vi "TestMeasure.vi"(7 "Samples":i32=5, 8 "error in (no error)":errorcluster, 11 "communication":i16(ring)=2 items=["USB - Nova2", "USB - Vega", "USB - USBI", "RS232", "GPIB"]) -> (0 "error out":errorcluster, 1 "variance":dbl format="%.2e", 2 "std deviation":dbl format="%.2e", 3 "mean":dbl format="%.4f")   [LabVIEW 2012]
doc: "PowerDemo.vi\nThe Demo enables power measurement and display results.\nVersion 1.00\nLast Updated 16 Mars 2005\n\nDemo Program Steps:\n \n1) The vi executes InitCom.vi to open the communication session.\nThe default is RS232,Port2,9600 bps and Address 10 for USB.\n\nYou have to select USB or RS232 Protocol and\nupdate these values for any change.\n\n2) The vi executes ConfMeasure.vi to Send \"FP\" (Force Power) to Device and \"SI\" (Send unIts) to receive the units\n\n3) The vi executes a loop of SendPower.vi to get measurements.\nWhen no Overrange value the vi add value to array for update\nstatistics values.\n\nIn case of Error:\nError Out contains the Error Number and the vi's name where the error occured.\n\nVISA Error Codes -10738077360 to -1073807231\nOphir Error Codes -1300 to 1340"
uses:
  <vilib>/Analysis/NI_AALBase.lvlib
panel:
  out "mean 2":dbl
  out "Units":string
  in  "Set Wavelength":string="275"
  out "Device Response 2":string="\r\n"
  out "Device Response":string="\r\n"
  out "Overrange":bool
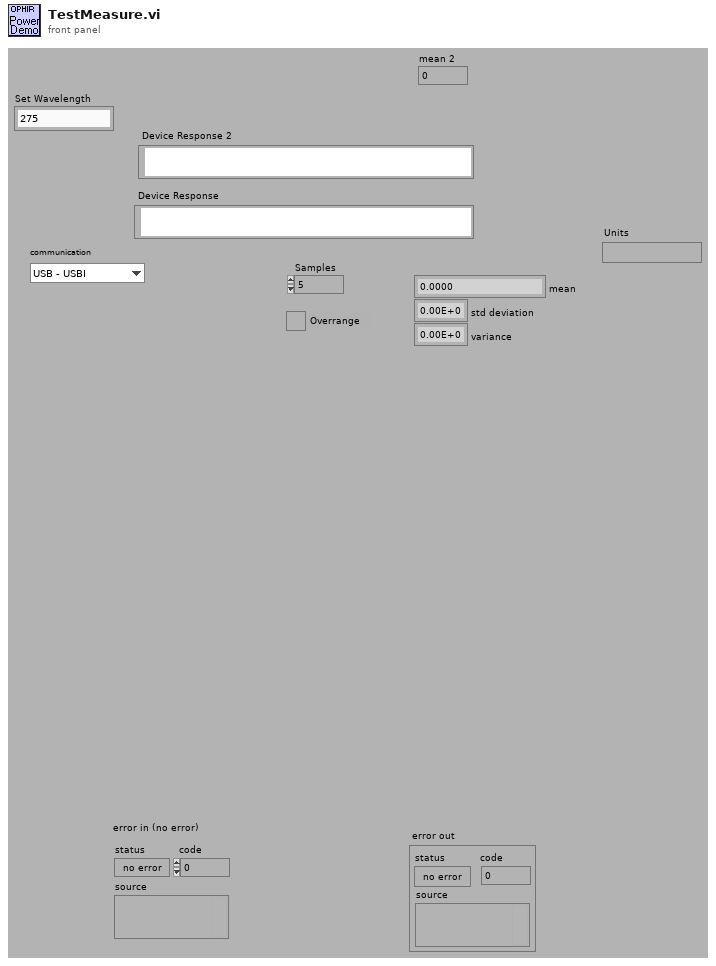
[diagram p1: front panel]
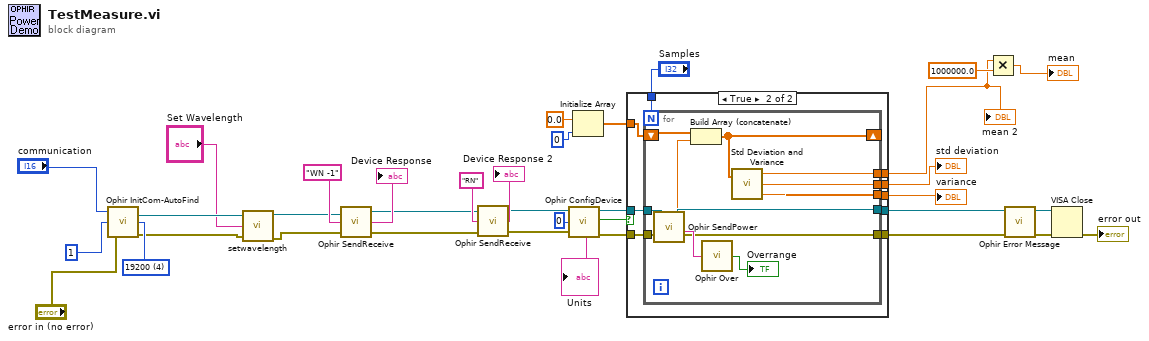
[diagram p0: block diagram]
diagram:
  w31 = i16 4 items=["300", "1200", "4800", "9600", "19200", "38400"] ("Baud Rate (3:9600)")
  n1 = call "Ophir InitCom-AutoFind.vi"("Baud Rate (3:9600)"=w31, "communication"="communication", "Port Number (default 2)"=i16 1, "error in (no error)"="error in (no error)") -> ("Dup Visa Session"=w7:refnum<visa-resource-name>, "error out"=w6:errorcluster)  [unwired: 2 out]
  n2 = call "setwavelength.vi"("Dup Visa Session"=w7, "Set Wavelength"="Set Wavelength", "error in (no error)"=w6) -> ("dup Visa Session"=w9:refnum<visa-resource-name>, "error out"=w8:errorcluster)  [unwired: 3 in]
  n3 = call "Ophir SendReceive.vi"("error in (no error)"=w8, "Command"="WN -1", "Visa Session"=w9) -> ("error out"=w11:errorcluster, "Frame Output"=→"Device Response":string, "dup Visa Session"=w13:refnum<visa-resource-name>)
  n4 = call "Ophir SendReceive.vi"("error in (no error)"=w11, "Command"="RN", "Visa Session"=w13) -> ("error out"=w10:errorcluster, "Frame Output"=→"Device Response 2":string, "dup Visa Session"=w12:refnum<visa-resource-name>)
  n5 = call "Ophir ConfigDevice.vi"("Visa Session"=w12, "Measure Choice (0:Power)"=u16 0, "error in (no error)"=w10) -> ("dup Visa Session"=w33:refnum<visa-resource-name>, "OK ?"=w34:bool, "Units"=→"Units":string, "error out"=w32:errorcluster)
  n6 = Initialize Array(0.0 ("element"), 0 ("dimension size")) -> (w21:dbl[])
  n7 = case shown="True" w34 {
    tunnel: w33 -> [w37 w47]
    tunnel: w32 -> [w38 w46]
    tunnel: [w37 w45] -> w28
    tunnel: [w38 w44] -> w25
    tunnel: "Samples" -> [_ w43]
    tunnel: w21 -> [_ w42]
    tunnel: [_ w41] -> w20
    tunnel: [_ w40] -> w19
    tunnel: [_ w39] -> w2
    frame False {
      # "Force Power Configuration failed"
    }
    frame True {
      n8 = for {
        N: w43 -> [_]
        tunnel: w47 -> [w59]
        tunnel: w46 -> [w58]
        tunnel: [w57] -> w45
        tunnel: [w54] -> w44
        shift-right: [w51] -> _
        shift-left: w42 -> [w53]
        tunnel: [w50] -> w39
        tunnel: [w49] -> w40
        tunnel: [w48] -> w41
        n9 = call "Ophir SendPower.vi"("Visa Session"=w59, "error in (no error)"=w58) -> ("dup Visa Session"=w57:refnum<visa-resource-name>, "Value Number"=w52:dbl, "Value String"=w56:string, "error out"=w54:errorcluster)
        n10 = Build Array (concatenate)(w53, w52) -> (w51:dbl[])
        n11 = call "Ophir Over.vi"("Value String"=w56) -> ("Overrange"=→"Overrange":bool)
        n12 = call <vilib>:"Std Deviation and Variance.vi"("X"=w51) -> ("mean"=w50:dbl, "standard deviation"=w49:dbl, "variance"=w48:dbl)  [unwired: 1 in]
      }
    }
  }
  "std deviation" <- w19
  "variance" <- w20
  "mean 2" <- w2
  n13 = Multiply(x=w2, y=1000000.0) -> (x*y=→"mean":dbl)
  n14 = call "Ophir Error Message.vi"("error in (no error)"=w25, "Visa Session"=w28) -> ("error out"=w26:errorcluster, "dup Visa Session"=w27:refnum<visa-resource-name>)  [unwired: 2 in, 2 out]
  n15 = VISA Close(VISA resource name=w27, error in (no error)=w26) -> (error out=→"error out":errorcluster)
